vi "modulo_2_de_comunicao_labview_unity.vi"(9 "number":i32, 10 "String":string, 11 "address":string) -> (2 "decimal integer string":string, 3 "concatenated string":string)   [LabVIEW 2017]
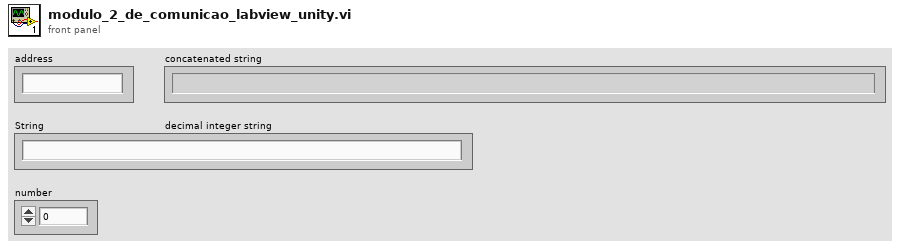
[diagram p1: front panel]
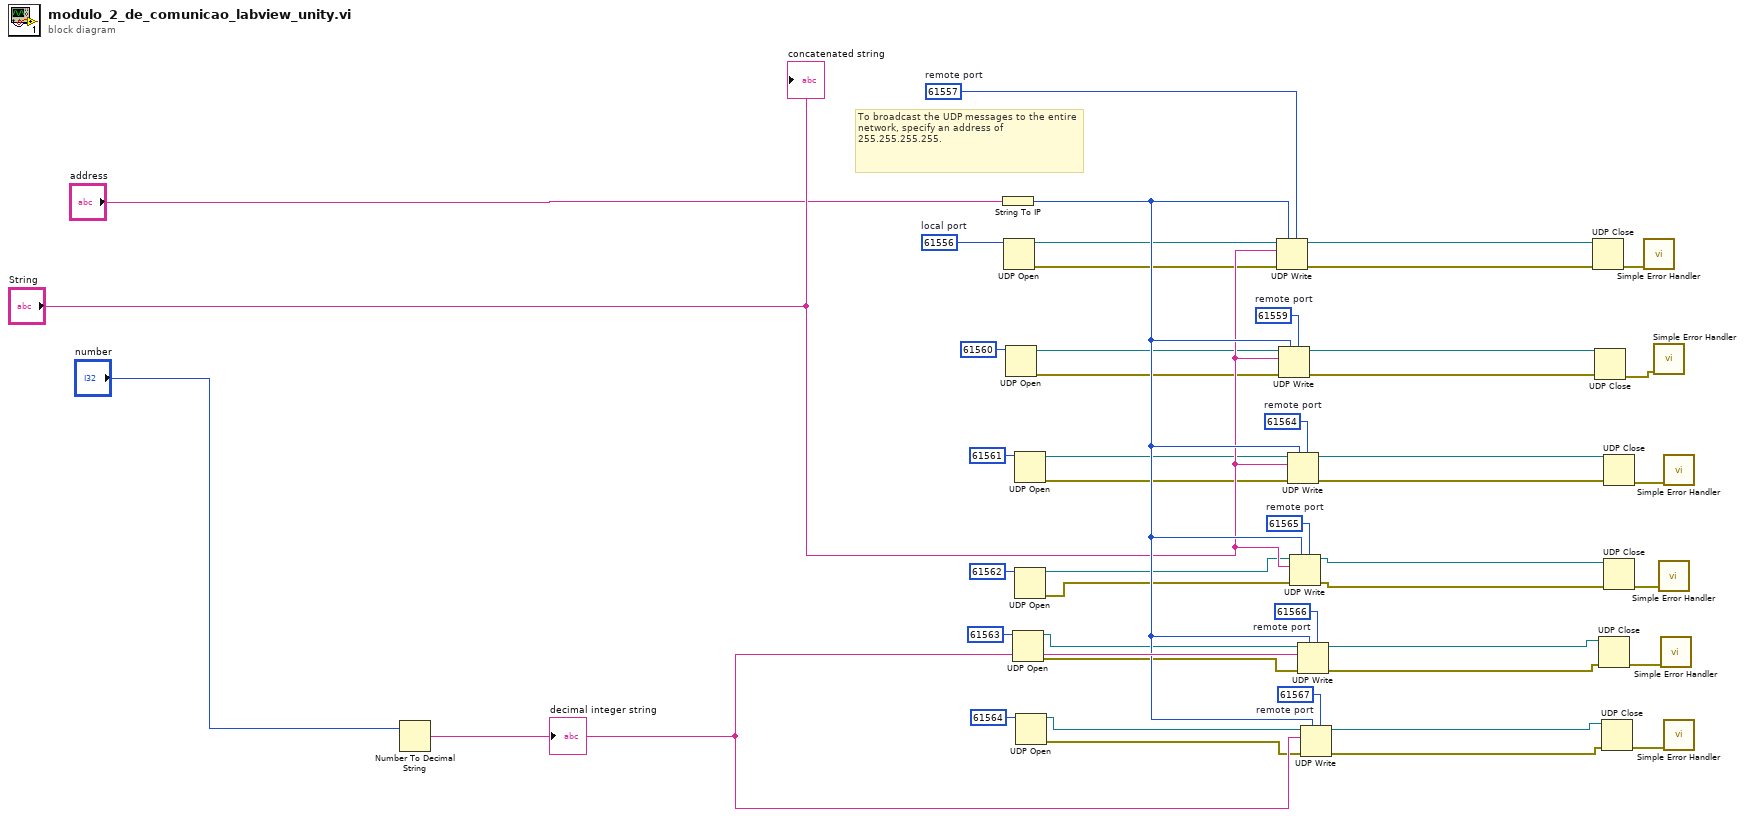
[diagram p0: block diagram]
diagram:
  w39 = u16 61567  # remote port
  w24 = u16 61566  # remote port
  w23 = u16 61565  # remote port
  w18 = u16 61564  # remote port
  w12 = u16 61559  # remote port
  w7 = u16 61557  # remote port
  w11 = u16 61556  # local port
  # "To broadcast the UDP messages to the entire network, specify an address of 255.255.255.255."
  n1 = Number To Decimal String(number="number") -> (decimal integer string=w46:string)  [unwired: 1 in]
  "decimal integer string" <- w46
  n2 = String To IP(1:"address") -> (0:w45:u32)
  n3 = UDP Open(11:w11) -> (port=w5:refnum<k16>, 0:w6:errorcluster)  [unwired: 4 in, 1 out]
  n4 = UDP Open(11:u16 61560 ("port")) -> (port=w10:refnum<k16>, 0:w13:errorcluster)  [unwired: 4 in, 1 out]
  n5 = UDP Open(11:u16 61563 ("port")) -> (port=w26:refnum<k16>, 0:w32:errorcluster)  [unwired: 4 in, 1 out]
  n6 = UDP Open(11:u16 61561 ("port")) -> (port=w17:refnum<k16>, 0:w19:errorcluster)  [unwired: 4 in, 1 out]
  n7 = UDP Open(11:u16 61562 ("port")) -> (port=w25:refnum<k16>, 0:w31:errorcluster)  [unwired: 4 in, 1 out]
  n8 = UDP Open(11:u16 61564 ("port")) -> (port=w40:refnum<k16>, 0:w43:errorcluster)  [unwired: 4 in, 1 out]
  n9 = UDP Write(address=w45, port or service name=w7, connection ID=w5, data in="String", 8:w6) -> (error out=w2:errorcluster, 3:w1:refnum<k16>)  [unwired: 1 in]
  n10 = UDP Write(address=w45, port or service name=w12, connection ID=w10, data in="String", 8:w13) -> (error out=w9:errorcluster, 3:w8:refnum<k16>)  [unwired: 1 in]
  n11 = UDP Write(address=w45, port or service name=w18, connection ID=w17, data in="String", 8:w19) -> (error out=w16:errorcluster, 3:w15:refnum<k16>)  [unwired: 1 in]
  n12 = UDP Write(address=w45, port or service name=w23, connection ID=w25, data in="String", 8:w31) -> (error out=w29:errorcluster, 3:w27:refnum<k16>)  [unwired: 1 in]
  n13 = UDP Write(address=w45, port or service name=w24, connection ID=w26, data in=w46, 8:w32) -> (error out=w30:errorcluster, 3:w28:refnum<k16>)  [unwired: 1 in]
  n14 = UDP Write(address=w45, port or service name=w39, connection ID=w40, data in=w46, 8:w43) -> (error out=w42:errorcluster, 3:w41:refnum<k16>)  [unwired: 1 in]
  n15 = UDP Close(connection ID=w1, 8:w2) -> (error out=w4:errorcluster)  [unwired: 1 out]
  n16 = UDP Close(connection ID=w8, 8:w9) -> (error out=w33:errorcluster)  [unwired: 1 out]
  n17 = UDP Close(connection ID=w28, 8:w30) -> (error out=w36:errorcluster)  [unwired: 1 out]
  n18 = UDP Close(connection ID=w41, 8:w42) -> (error out=w44:errorcluster)  [unwired: 1 out]
  n19 = UDP Close(connection ID=w15, 8:w16) -> (error out=w34:errorcluster)  [unwired: 1 out]
  n20 = UDP Close(connection ID=w27, 8:w29) -> (error out=w35:errorcluster)  [unwired: 1 out]
  n21 = call <vilib>:"Simple Error Handler.vi"("error in (no error)"=w4) -> ()  [unwired: 4 in, 5 out]
  n22 = call <vilib>:"Simple Error Handler.vi"("error in (no error)"=w33) -> ()  [unwired: 4 in, 5 out]
  n23 = call <vilib>:"Simple Error Handler.vi"("error in (no error)"=w35) -> ()  [unwired: 4 in, 5 out]
  n24 = call <vilib>:"Simple Error Handler.vi"("error in (no error)"=w36) -> ()  [unwired: 4 in, 5 out]
  n25 = call <vilib>:"Simple Error Handler.vi"("error in (no error)"=w34) -> ()  [unwired: 4 in, 5 out]
  n26 = call <vilib>:"Simple Error Handler.vi"("error in (no error)"=w44) -> ()  [unwired: 4 in, 5 out]
  "concatenated string" <- "String"
